vi "shutdown.vi"(7 "references":T1, 8 "error in (no error)":errorcluster) -> (0 "error out":errorcluster)   [LabVIEW 2015, in "repub-dvr_nre.lvlib"]
doc: "This VI can be used to shutdown the module. Note that it doesn't need to use the input queue since it's destroying/closing references rather than creating them. Once complete, it sets the initialize flag to false."
uses:
  repub-dvr_nre.lvlib
  _controls/references.ctl
  private/_controls/input.ctl
  private/_controls/input_command.ctl
  private/_controls/output.ctl
  private/_controls/data.ctl
  _controls/configuration.ctl
  _controls/change.ctl
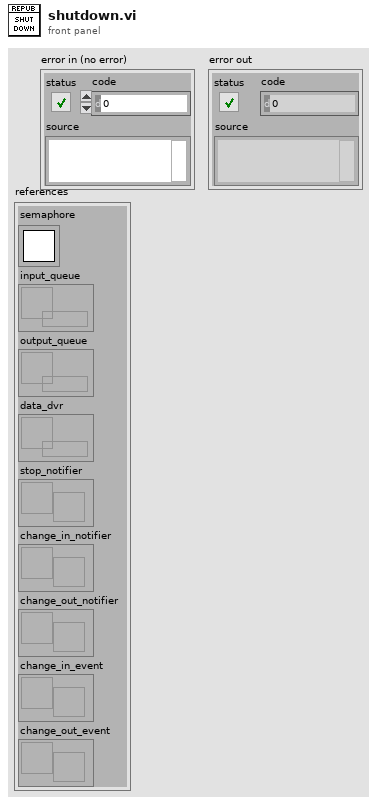
[diagram p1: front panel]
types:
  T1 = typedef "repub-dvr_nre.lvlib/references.ctl" = cluster{"semaphore":T2, "input_queue":refnum<queue>, "output_queue":refnum<queue>, "data_dvr":refnum<data-value>, "stop_notifier":refnum<notifier>, "change_in_notifier":refnum<notifier>, "change_out_notifier":refnum<notifier>, "change_in_event":refnum<user-event>, "change_out_event":refnum<user-event>}
  T2 = typedef "Semaphore RefNum" = refnum<k1>
  T3 = typedef "repub-dvr_nre.lvlib/data.ctl" = cluster{"configuration":T4, "working":cluster{"initialized":bool}}
  T4 = typedef "repub-dvr_nre.lvlib/configuration.ctl" = cluster{dbl}
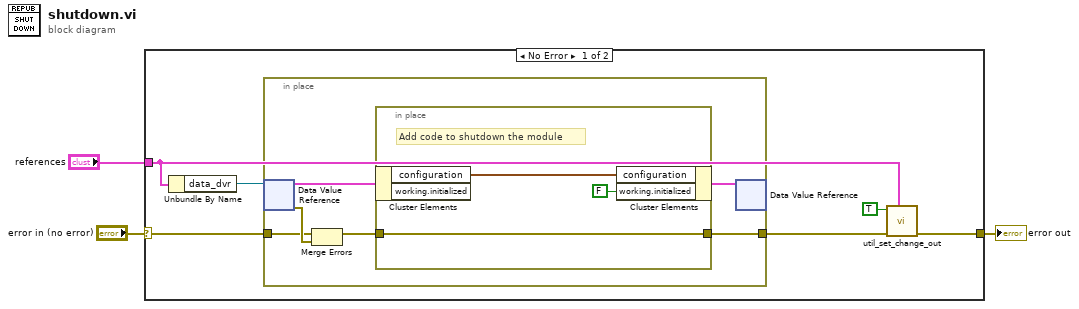
[diagram p0: block diagram]
diagram:
  n1 = case shown="No Error" "error in (no error)" {
    selector: "error in (no error)" -> [w8 w19]
    tunnel: [w5 w19] -> w2
    tunnel: "references" -> [w6 _]
    frame No Error {
      n2 = Unbundle By Name(w6) -> ("data_dvr"=w9:refnum<data-value>)
      n3 = in-place {
        in-place-border: [w10] -> w4
        in-place-border: w8 -> [w14]
        n4 = in-place-dvr #1(w9) -> (w13:T3, w15:errorcluster)
        n5 = Merge Errors(w14, w15) -> (w11:errorcluster)
        n6 = in-place {
          in-place-border: w11 -> [w17]
          in-place-border: [w17] -> w10
          # "Add code to shutdown the module"
          n7 = in-place-cluster #2(w13) -> ("configuration"=w18:T4)  [unwired: 1 out]
          n8 = in-place-cluster #2("configuration"=w18, "working.initialized"=FALSE) -> (w12:T3)
        }
        n9 = in-place-dvr #1(w12) -> ()  [unwired: 2 out]
      }
      n10 = call "util_set_change_out.vi"("references"=w6, "error in (no error)"=w4, "change"=TRUE) -> ("error out"=w5:errorcluster)  [unwired: 8 in]
    }
    frame Error {
    }
  }
  "error out" <- w2
